vi "cobaaa.vi"() -> ()   [LabVIEW 2015, in "Untitled Library 2.lvlib"]
uses:
  Untitled Library 2.lvlib
  <vilib>/rvi/Emulation/niFpgaGetClockAttributes.vi
  <vilib>/rvi/Emulation/niFpgaSctlEmulationGetInTimedLoop.vi
  <vilib>/rvi/Emulation/niFpgaEmulationReportErrorSimple.vi
  <vilib>/rvi/eio/common/nirviEmuTemplateMethod_errors.vi
  <vilib>/rvi/Emulation/niFpgaCriticalErrorInLSC.vi
  <vilib>/eio/EIONode/EIONode.xnode
panel:
  out "LED 2":bool
  out "FPGA I/O Out 2":refnum<k21>
  in  "Count(Ticks)":u32
  in  "y":u16
  in  "x":u16
  in  "STOP":bool
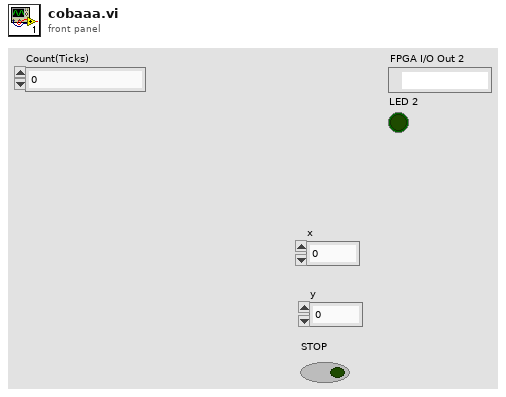
[diagram p1: front panel]
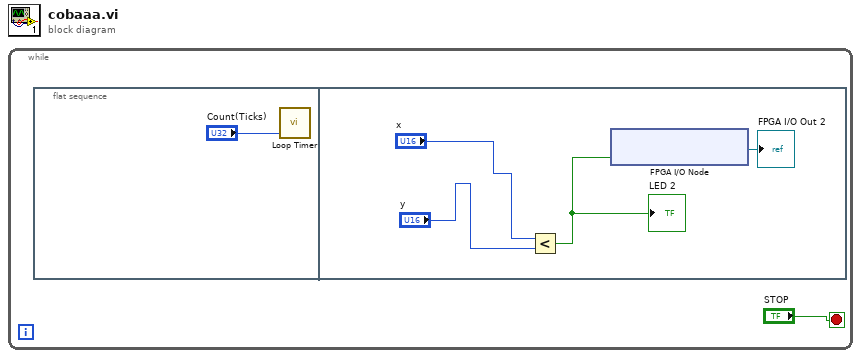
[diagram p0: block diagram]
diagram:
  n1 = while {
    stop <- "STOP" stop-if-true
    n2 = flat-sequence {
      frame #0 {
        n3 = call "Loop Timer"("Count(Ticks)"="Count(Ticks)") -> ()  [unwired: 1 out]
      }
      frame #1 {
        n4 = Less?(x="x", y="y") -> (x < y?=w5:bool)
        "LED 2" <- w5
        n5 = xnode "FPGA I/O Node"("ConnectorB/DIO8"=w5) -> ("FPGA I/O Out"=→"FPGA I/O Out 2":refnum<k21>)  [unwired: 1 in]
      }
    }
  }
